vi "Select_bool.vi"(8 "False":T1, 10 "Input":T1, 11 "True":T1) -> (2 "output cluster":T1)   [LabVIEW 2017]
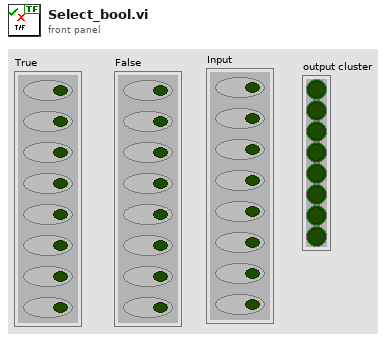
[diagram p1: front panel]
types:
  T1 = cluster{bool, bool, bool, bool, bool, bool, bool, bool}
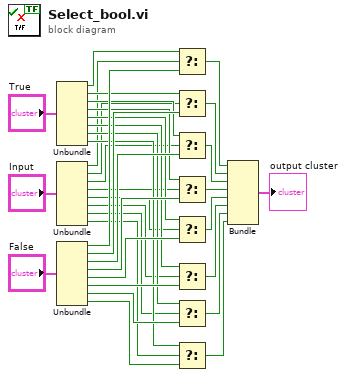
[diagram p0: block diagram]
diagram:
  n1 = Unbundle("True") -> (w13:bool, w14:bool, w15:bool, w16:bool, w17:bool, w18:bool, w19:bool, w20:bool)
  n2 = Unbundle("Input") -> (w11:bool, w10:bool, w9:bool, w8:bool, w7:bool, w6:bool, w5:bool, w4:bool)
  n3 = Unbundle("False") -> (w21:bool, w22:bool, w23:bool, w24:bool, w25:bool, w26:bool, w27:bool, w28:bool)
  n4 = Select(t=w13, s=w11, f=w21) -> (s? t:f=w36:bool)
  n5 = Select(t=w14, s=w10, f=w22) -> (s? t:f=w35:bool)
  n6 = Select(t=w15, s=w9, f=w23) -> (s? t:f=w34:bool)
  n7 = Select(t=w16, s=w8, f=w24) -> (s? t:f=w33:bool)
  n8 = Select(t=w17, s=w7, f=w25) -> (s? t:f=w32:bool)
  n9 = Select(t=w18, s=w6, f=w26) -> (s? t:f=w31:bool)
  n10 = Select(t=w19, s=w5, f=w27) -> (s? t:f=w30:bool)
  n11 = Select(t=w20, s=w4, f=w28) -> (s? t:f=w29:bool)
  n12 = Bundle(w36, w35, w34, w33, w32, w31, w30, w29) -> (→"output cluster":T1)  [unwired: 1 in]
